vi "MultiAxisControl.vi"() -> ()   [LabVIEW 2020]
uses:
  <vilib>/Utility/config.llb/Read Key (I32).vi
  <vilib>/Utility/config.llb/Read Key (String).vi
  Recipe.vi
  <vilib>/Utility/config.llb/Write Key (I32).vi
  <vilib>/Utility/config.llb/Write Key (String).vi
  ConnectionData.vi
  ConnectionData_Write.vi
  <vilib>/Utility/config.llb/NI_LVConfig.lvlib
  SMCD14_lib.lvlib
panel:
  in  "StopAppBtn":bool caption="Close"
  in  "Recipe":bool
  in  "Chart":bool
  in  "DisconnectBtn":bool
  in  "ConnectBtn":bool
  out "AxesCount":i32=6
  out "AxisControlSubPanelsArray":refnum<vi>[](array[refnum])
  in  "error in (no error)":errorcluster
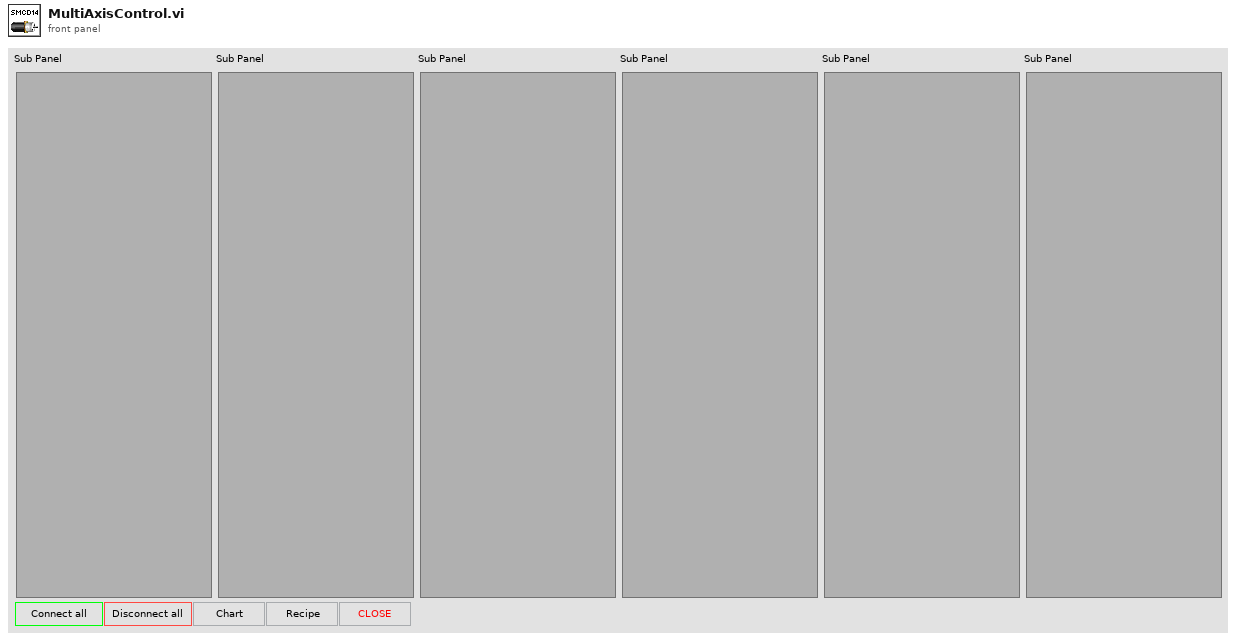
[diagram p1: front panel]
types:
  T1 = enum32{"Invalid", "Standard", "Closed", "Hidden", "Minimized", "Maximized"}
  T2 = typedef "NI_LVConfig.lvlib/Config Data RefNum.ctl" = refnum<k1>
  T3 = typedef "LVRectTypeDef.ctl" = cluster{"Left":i16, "Top":i16, "Right":i16, "Bottom":i16}
  T4 = enum32{"Bad", "Idle", "Run top level", "Running"}
  T5 = typedef "SMCD14_lib.lvlib/ConnectionData_typedef.ctl" = cluster{"DeviceIDCtrl":u16, "ProtocolCtrl":enum16{"Modbus RTU", "Modbus TCP", ""}, "COMportCtrl":refnum<visa-resource-name>, "IPCtrl":string, "serial master instance":refnum<class "Modbus Master.lvclass">, "ConnectionStatusIndicator":bool}
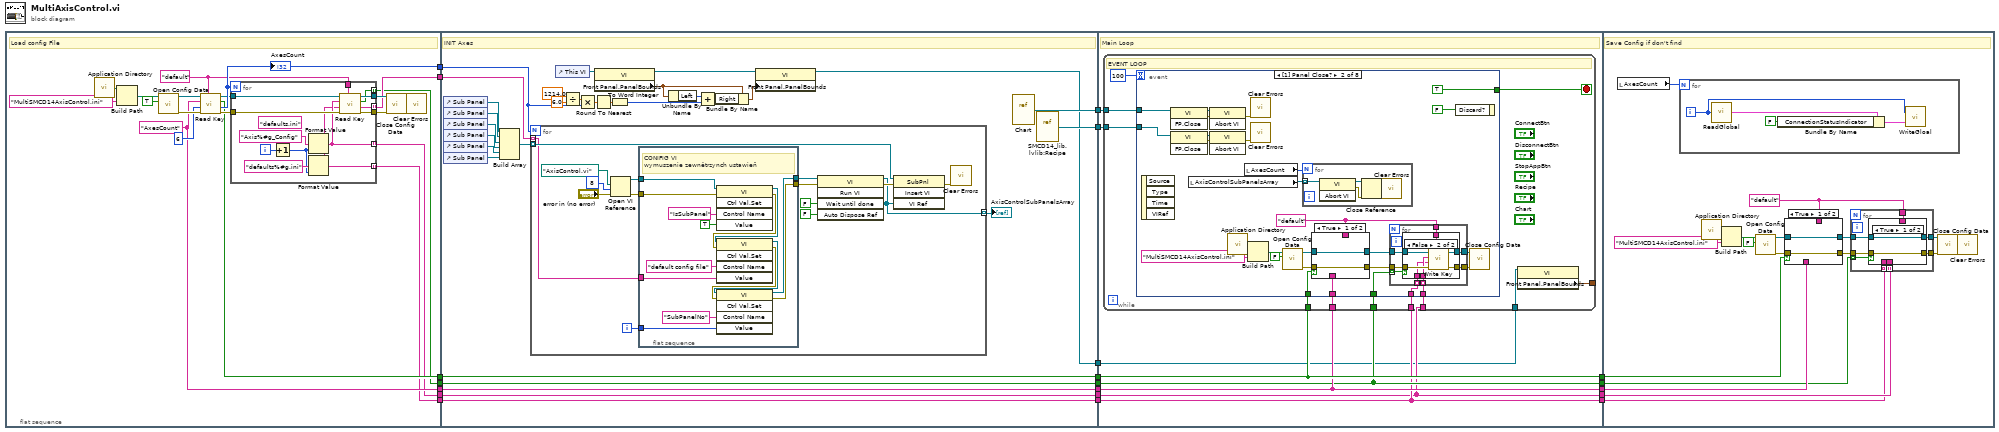
[diagram p0: block diagram]
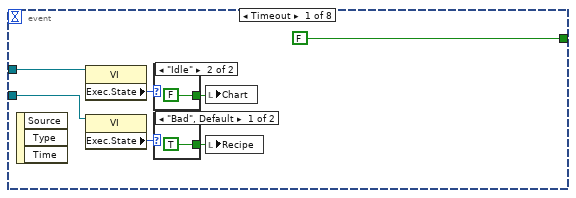
[diagram p2: hidden frame]
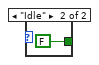
[diagram p3: hidden frame]
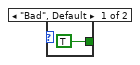
[diagram p4: hidden frame]
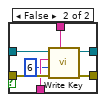
[diagram p6: hidden frame]
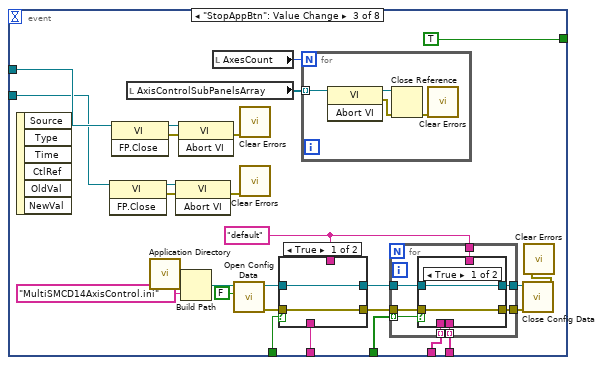
[diagram p7: hidden frame]
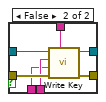
[diagram p8: hidden frame]
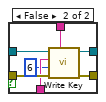
[diagram p9: hidden frame]
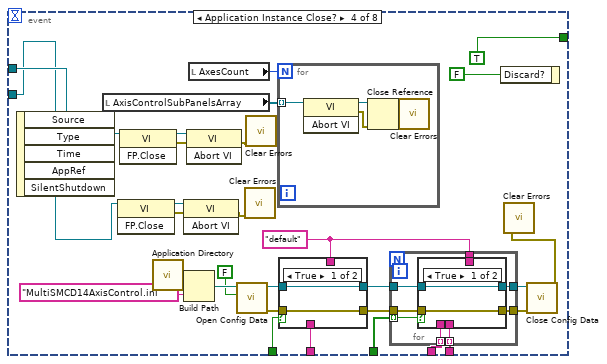
[diagram p10: hidden frame]
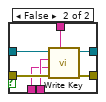
[diagram p11: hidden frame]
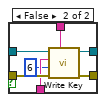
[diagram p12: hidden frame]
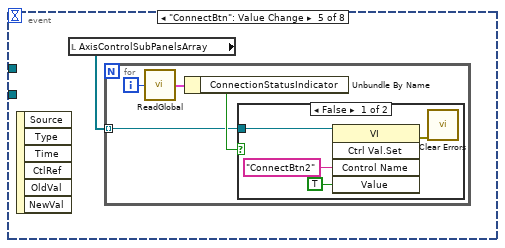
[diagram p13: hidden frame]
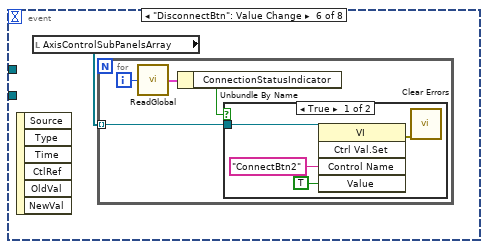
[diagram p15: hidden frame]
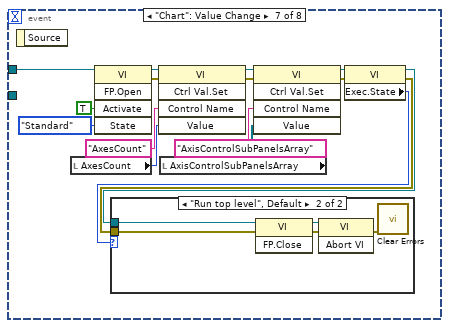
[diagram p17: hidden frame]
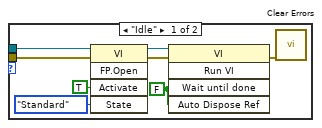
[diagram p18: hidden frame]
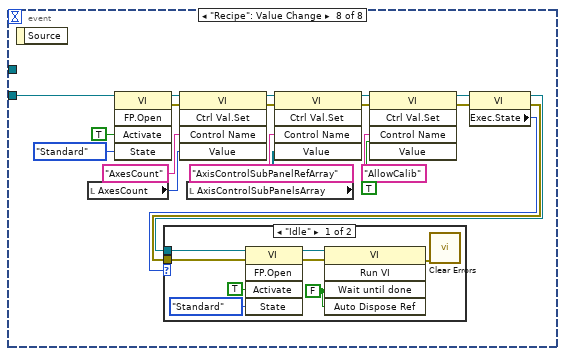
[diagram p19: hidden frame]
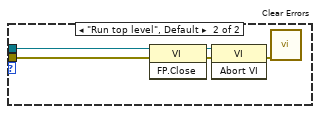
[diagram p20: hidden frame]
diagram:
  n1 = flat-sequence {
    tunnel: [w33] -> w20
    tunnel: [w27] -> w19
    tunnel: [w26] -> w18
    tunnel: [w25] -> w17
    tunnel: [w24] -> w12
    tunnel: [w23] -> w11
    tunnel: [w22] -> w10
    tunnel: w20 -> [w68]
    tunnel: w19 -> [w80]
    tunnel: w18 -> [w79]
    tunnel: w17 -> [w78]
    tunnel: [w79] -> w16
    tunnel: [w78] -> w15
    tunnel: w12 -> [w77]
    tunnel: w11 -> [w76]
    tunnel: w10 -> [w75]
    tunnel: [w77] -> w9
    tunnel: [w76] -> w8
    tunnel: [w75] -> w7
    tunnel: [w74] -> w3
    tunnel: [w73] -> w2
    tunnel: [w54] -> w1
    tunnel: w16 -> [w119]
    tunnel: w15 -> [w117]
    tunnel: [w119] -> w14
    tunnel: [w117] -> w13
    tunnel: w9 -> [w118]
    tunnel: w8 -> [w115]
    tunnel: w7 -> [w116]
    tunnel: [w118] -> w6
    tunnel: [w115] -> w5
    tunnel: [w116] -> w4
    tunnel: w3 -> [w114]
    tunnel: w2 -> [w113]
    tunnel: w1 -> [w112]
    tunnel: w14 -> [w407]
    tunnel: w13 -> [w404]
    tunnel: w6 -> [w408]
    tunnel: w5 -> [w406]
    tunnel: w4 -> [w405]
    frame #0 {
      w24 = "AxesCount" ("key")
      w30 = "default" ("section")
      # "Load config File"
      n2 = call <vilib>:"Application Directory.vi"() -> ("Application Directory"=w39:path)
      n3 = Build Path(base path=w39, name or relative path="MultiSMCD14AxisControl.ini") -> (appended path=w35:path)
      n4 = call <vilib>:"Open Config Data.vi"("create file if necessary (T)"=TRUE, "configuration file path"=w35) -> ("error out"=w36:errorcluster, "refnum"=w37:T2)  [unwired: 7 in, 1 out]
      n5 = call-poly <vilib>:"Read Key.vi"("section"=w30, "error in (no error)"=w36, "default value"=6, "key"=w24, "refnum"=w37) -> ("error out"=w31:errorcluster, "value"=w33:i32, "found?"=w26:bool, "refnum out"=w32:T2)  [unwired: 3 in]
      "AxesCount" <- w33
      n6 = for {
        N: w33 -> [_]
        tunnel: w32 -> [w51]
        tunnel: w31 -> [w50]
        tunnel: [w49] -> w29
        tunnel: [w48] -> w28
        tunnel: [w47] -> w27 mode=indexing
        tunnel: w30 -> [w46]
        tunnel: [w43] -> w25 mode=indexing
        tunnel: [w42] -> w23 mode=indexing
        tunnel: [w41] -> w22 mode=indexing
        i -> [w53]
        (unwired) "defaults.ini" ("default value")
        n7 = Increment(x=w53) -> (x+1=w44:i32)
        n8 = Format Value(format string="Axis%#g_Config" ("key"), value (0)=w44) -> (output string=w42:string)  [unwired: 1 in]
        n9 = Format Value(format string="defaults%#g.ini" ("default value"), value (0)=w44) -> (output string=w41:string)  [unwired: 1 in]
        n10 = call-poly <vilib>:"Read Key.vi"("section"=w46, "error in (no error)"=w50, "default value"=w41, "key"=w42, "refnum"=w51) -> ("error out"=w48:errorcluster, "value"=w47:string, "found?"=w43:bool, "refnum out"=w49:T2)  [unwired: 3 in]
      }
      n11 = call <vilib>:"Close Config Data.vi"("error in (no error)"=w28, "refnum"=w29) -> ("error out"=w21:errorcluster)  [unwired: 8 in, 1 out]
      n12 = call <vilib>:"Clear Errors.vi"("error in (no error)"=w21) -> ()  [unwired: 5 in, 2 out]
    }
    frame #1 {
      # "INIT Axes"
      n13 = control-ref of="Sub Panel"() -> (w60:refnum<vi>)
      n14 = control-ref of="Sub Panel"() -> (w59:refnum<vi>)
      n15 = control-ref of="Sub Panel"() -> (w58:refnum<vi>)
      n16 = control-ref of="Sub Panel"() -> (w57:refnum<vi>)
      n17 = control-ref of="Sub Panel"() -> (w56:refnum<vi>)
      n18 = control-ref of="Sub Panel"() -> (w55:refnum<vi>)
      n19 = Build Array(w60, w59, w58, w57, w56, w55) -> (w81:refnum<vi>[])
      n20 = for {
        N: w68 -> [_]
        tunnel: w81 -> [w94] mode=indexing
        tunnel: [w84] -> w82 mode=indexing
        tunnel: w80 -> [w86] mode=indexing
        i -> [w85]
        n21 = Open VI Reference(vi path=path "AxisControl.vi", options=8, error in (no error)="error in (no error)") -> (vi reference=w88:refnum<vi>, error out=w87:errorcluster)  [unwired: 3 in]
        n22 = flat-sequence {
          tunnel: w88 -> [w109]
          tunnel: [w100] -> w95
          tunnel: w87 -> [w108]
          tunnel: [w101] -> w93
          tunnel: w86 -> [w104]
          tunnel: w85 -> [w103]
          frame #0 {
            # "CONIFIG VI\nwymuszenie zewnêtrzynch ustawieñ"
            n23 = invoke class="VI" method="Ctrl Val.Set"(reference=w109, error in=w108, "Control Name"="IsSubPanel", "Value"=TRUE) -> (reference out=w106:refnum<vi>, error out=w105:errorcluster)  [unwired: 1 in, 3 out]
            n24 = invoke class="VI" method="Ctrl Val.Set"(reference=w106, error in=w105, "Control Name"="default config file", "Value"=w104) -> (reference out=w99:refnum<vi>, error out=w98:errorcluster)  [unwired: 1 in, 3 out]
            n25 = invoke class="VI" method="Ctrl Val.Set"(reference=w99, error in=w98, "Control Name"="SubPanelNo", "Value"=w103) -> (reference out=w101:refnum<vi>, error out=w100:errorcluster)  [unwired: 1 in, 3 out]
          }
        }
        n26 = invoke class="VI" method="Run VI"(reference=w93, error in=w95, "Wait until done"=FALSE ("Wait Until Done"), "Auto Dispose Ref"=FALSE ("Auto Dispose Reference")) -> (reference out=w84:refnum<vi>, error out=w92:errorcluster)  [unwired: 1 in, 3 out]
        n27 = invoke class="SubPnl" method="Insert VI"(reference=w94, error in=w92, "VI Ref"=w84) -> (error out=w83:errorcluster)  [unwired: 1 in, 3 out]
        n28 = call <vilib>:"Clear Errors.vi"("error in (no error)"=w83) -> ()  [unwired: 5 in, 2 out]
      }
      "AxisControlSubPanelsArray" <- w82
      n29 = control-ref of="This VI"() -> (w72:refnum<vi>)
      n30 = Divide(x=1214.0, y=6.0) -> (x/y=w69:dbl)
      n31 = Multiply(x=w69, y=w68) -> (x*y=w67:dbl)
      n32 = Round To Nearest(number=w67) -> (nearest integer value=w66:dbl)
      n33 = property class="VI"(reference=w72) -> ("Front Panel.PanelBounds"=w64:T3)  [unwired: 1 in, 2 out]
      n34 = To Word Integer(number=w66) -> (16bit integer=w62:i16)
      n35 = Unbundle By Name(w64) -> ("Left"=w61:i16)
      n36 = Add(x=w61, y=w62) -> (x+y=w63:i16)
      n37 = Bundle By Name(cluster=w64, "Right"=w63) -> (w65:T3)
      n38 = property class="VI"(reference=w72, "Front Panel.PanelBounds"=w65) -> (reference out=w54:refnum<vi>)  [unwired: 1 in, 1 out]
      n39 = vi-ref "Chart.vi"() -> (w74:refnum<vi>)
      n40 = vi-ref "SMCD14_lib.lvlib:Recipe.vi"() -> (w73:refnum<vi>)
    }
    frame #2 {
      # "Main Loop"
      n41 = while {
        tunnel: w119 -> [w128]
        tunnel: w118 -> [w127]
        tunnel: w117 -> [w126]
        tunnel: w116 -> [w125]
        tunnel: w115 -> [w124]
        tunnel: w114 -> [w123]
        tunnel: w113 -> [w122]
        tunnel: [w121] -> _
        tunnel: w112 -> [w120]
        stop <- w129 stop-if-true
        # "EVENT LOOP"
        n42 = event shown="[1] Panel Close?" {
          selector: _ -> [_ _ _ _ _ _ _ _]
          dyn-events: _ -> [_ _ _ _ _ _ _ _]
          timeout: 100 -> [_ _ _ _ _ _ _ _]
          tunnel: [FALSE ("Discard?") TRUE ("Discard?") TRUE ("Discard?") TRUE ("Discard?") _ _ _ _] -> w129
          tunnel: w128 -> [_ w154 w213 w275 _ _ _ _]
          tunnel: w127 -> [_ w153 w212 w274 _ _ _ _]
          tunnel: w126 -> [_ w152 w211 w273 _ _ _ _]
          tunnel: w125 -> [_ w151 w210 w272 _ _ _ _]
          tunnel: w124 -> [_ w150 w209 w271 _ _ _ _]
          tunnel: w123 -> [w136 w149 w208 w262 _ _ w344 _]
          tunnel: w122 -> [w132 w146 w205 w261 _ _ _ w371]
          event Timeout {
            n43 = event-data() -> ()  [unwired: 1 in, 3 out]
            n44 = property class="VI"(reference=w136) -> ("Exec.State"=w135:T4)  [unwired: 1 in, 2 out]
            n45 = property class="VI"(reference=w132) -> ("Exec.State"=w133:T4)  [unwired: 1 in, 2 out]
            n46 = case shown="\"Idle\"" w135 {
              tunnel: [TRUE ("Chart") FALSE ("Chart")] -> w134
              frame "Bad", Default {
              }
              frame "Idle" {
              }
            }
            n47 = case shown="\"Bad\", Default" w133 {
              tunnel: [TRUE ("Chart") FALSE ("Chart")] -> w131
              frame "Bad", Default {
              }
              frame "Idle" {
              }
            }
            n48 = local write "Chart"(w134) -> ()
            n49 = local write "Recipe"(w131) -> ()
          }
          event Panel Close? {
            w159 = "default" ("section")
            n50 = event-data() -> ()  [unwired: 1 in, 4 out]
            n51 = invoke class="VI" method="FP.Close"(reference=w149) -> (reference out=w148:refnum<vi>, error out=w145:errorcluster)  [unwired: 2 in, 1 out]
            n52 = invoke class="VI" method="FP.Close"(reference=w146) -> (reference out=w147:refnum<vi>, error out=w144:errorcluster)  [unwired: 2 in, 1 out]
            n53 = local read "AxisControlSubPanelsArray"() -> (w169:refnum<vi>[])
            n54 = invoke class="VI" method="Abort VI"(reference=w148, error in=w145) -> (error out=w143:errorcluster)  [unwired: 1 in, 2 out]
            n55 = invoke class="VI" method="Abort VI"(reference=w147, error in=w144) -> (error out=w142:errorcluster)  [unwired: 1 in, 2 out]
            n56 = call <vilib>:"Application Directory.vi"() -> ("Application Directory"=w162:path)
            n57 = local read "AxesCount"() -> (w167:i32)
            n58 = Build Path(base path=w162, name or relative path="MultiSMCD14AxisControl.ini") -> (appended path=w163:path)
            n59 = call <vilib>:"Clear Errors.vi"("error in (no error)"=w143) -> ()  [unwired: 5 in, 2 out]
            n60 = call <vilib>:"Clear Errors.vi"("error in (no error)"=w142) -> ()  [unwired: 5 in, 2 out]
            n61 = call <vilib>:"Open Config Data.vi"("create file if necessary (T)"=FALSE, "configuration file path"=w163) -> ("error out"=w165:errorcluster, "refnum"=w164:T2)  [unwired: 7 in, 1 out]
            n62 = for {
              N: w167 -> [_]
              tunnel: w169 -> [w199] mode=indexing
              n63 = invoke class="VI" method="Abort VI"(reference=w199) -> (reference out=w198:refnum<vi>, error out=w197:errorcluster)  [unwired: 2 in, 1 out]
              n64 = Close Reference(reference=w198, error in (no error)=w197) -> (error out=w196:errorcluster)
              n65 = call <vilib>:"Clear Errors.vi"("error in (no error)"=w196) -> ()  [unwired: 5 in, 2 out]
            }
            n66 = case shown="True" w154 {
              tunnel: [w187 w195] -> w157
              tunnel: [w188 w194] -> w158
              tunnel: w165 -> [w187 w193]
              tunnel: w164 -> [w188 w192]
              tunnel: w153 -> [_ w191]
              tunnel: w159 -> [_ w189]
              frame True {
              }
              frame False {
                n67 = call-poly <vilib>:"Write Key.vi"("section"=w189, "error in (no error)"=w193, "value"=6, "key"=w191, "refnum"=w192) -> ("error out"=w195:errorcluster, "refnum out"=w194:T2)  [unwired: 4 in, 1 out]
              }
            }
            n68 = for {
              tunnel: w150 -> [w177] mode=indexing
              tunnel: w151 -> [w176] mode=indexing
              tunnel: w152 -> [w170] mode=indexing
              tunnel: w159 -> [w175]
              tunnel: w158 -> [w174]
              tunnel: w157 -> [w173]
              tunnel: [w172] -> w156
              tunnel: [w171] -> w155
              n69 = case shown="False" w170 {
                tunnel: [w178 w186] -> w171
                tunnel: [w179 w185] -> w172
                tunnel: w173 -> [w178 w184]
                tunnel: w174 -> [w179 w183]
                tunnel: w177 -> [_ w182]
                tunnel: w175 -> [_ w181]
                tunnel: w176 -> [_ w180]
                frame True {
                }
                frame False {
                  n70 = call-poly <vilib>:"Write Key.vi"("section"=w181, "error in (no error)"=w184, "value"=w180, "key"=w182, "refnum"=w183) -> ("error out"=w186:errorcluster, "refnum out"=w185:T2)  [unwired: 4 in, 1 out]
                }
              }
            }
            n71 = event-data("Discard?"=FALSE) -> ()  [unwired: 1 in, 1 out]
            n72 = call <vilib>:"Close Config Data.vi"("error in (no error)"=w155, "refnum"=w156) -> ()  [unwired: 8 in, 2 out]
          }
          event "StopAppBtn": Value Change {
            w218 = "default" ("section")
            n73 = event-data() -> ()  [unwired: 1 in, 6 out]
            n74 = invoke class="VI" method="FP.Close"(reference=w205) -> (reference out=w206:refnum<vi>, error out=w203:errorcluster)  [unwired: 2 in, 1 out]
            n75 = invoke class="VI" method="FP.Close"(reference=w208) -> (reference out=w207:refnum<vi>, error out=w204:errorcluster)  [unwired: 2 in, 1 out]
            n76 = local read "AxisControlSubPanelsArray"() -> (w227:refnum<vi>[])
            n77 = call <vilib>:"Application Directory.vi"() -> ("Application Directory"=w221:path)
            n78 = invoke class="VI" method="Abort VI"(reference=w206, error in=w203) -> (error out=w202:errorcluster)  [unwired: 1 in, 2 out]
            n79 = invoke class="VI" method="Abort VI"(reference=w207, error in=w204) -> (error out=w201:errorcluster)  [unwired: 1 in, 2 out]
            n80 = Build Path(base path=w221, name or relative path="MultiSMCD14AxisControl.ini") -> (appended path=w222:path)
            n81 = local read "AxesCount"() -> (w226:i32)
            n82 = call <vilib>:"Open Config Data.vi"("create file if necessary (T)"=FALSE, "configuration file path"=w222) -> ("error out"=w224:errorcluster, "refnum"=w223:T2)  [unwired: 7 in, 1 out]
            n83 = call <vilib>:"Clear Errors.vi"("error in (no error)"=w201) -> ()  [unwired: 5 in, 2 out]
            n84 = call <vilib>:"Clear Errors.vi"("error in (no error)"=w202) -> ()  [unwired: 5 in, 2 out]
            n85 = case shown="True" w213 {
              tunnel: [w245 w253] -> w216
              tunnel: [w246 w252] -> w217
              tunnel: w224 -> [w245 w251]
              tunnel: w223 -> [w246 w250]
              tunnel: w212 -> [_ w249]
              tunnel: w218 -> [_ w247]
              frame True {
              }
              frame False {
                n86 = call-poly <vilib>:"Write Key.vi"("section"=w247, "error in (no error)"=w251, "value"=6, "key"=w249, "refnum"=w250) -> ("error out"=w253:errorcluster, "refnum out"=w252:T2)  [unwired: 4 in, 1 out]
              }
            }
            n87 = for {
              N: w226 -> [_]
              tunnel: w227 -> [w257] mode=indexing
              n88 = invoke class="VI" method="Abort VI"(reference=w257) -> (reference out=w256:refnum<vi>, error out=w255:errorcluster)  [unwired: 2 in, 1 out]
              n89 = Close Reference(reference=w256, error in (no error)=w255) -> (error out=w254:errorcluster)
              n90 = call <vilib>:"Clear Errors.vi"("error in (no error)"=w254) -> ()  [unwired: 5 in, 2 out]
            }
            n91 = for {
              tunnel: w209 -> [w235] mode=indexing
              tunnel: w210 -> [w234] mode=indexing
              tunnel: w211 -> [w228] mode=indexing
              tunnel: w218 -> [w233]
              tunnel: w217 -> [w232]
              tunnel: w216 -> [w231]
              tunnel: [w230] -> w215
              tunnel: [w229] -> w214
              n92 = case shown="True" w228 {
                tunnel: [w236 w244] -> w229
                tunnel: [w237 w243] -> w230
                tunnel: w231 -> [w236 w242]
                tunnel: w232 -> [w237 w241]
                tunnel: w235 -> [_ w240]
                tunnel: w233 -> [_ w239]
                tunnel: w234 -> [_ w238]
                frame True {
                }
                frame False {
                  n93 = call-poly <vilib>:"Write Key.vi"("section"=w239, "error in (no error)"=w242, "value"=w238, "key"=w240, "refnum"=w241) -> ("error out"=w244:errorcluster, "refnum out"=w243:T2)  [unwired: 4 in, 1 out]
                }
              }
            }
            n94 = call <vilib>:"Close Config Data.vi"("error in (no error)"=w214, "refnum"=w215) -> ("error out"=w200:errorcluster)  [unwired: 8 in, 1 out]
            n95 = call <vilib>:"Clear Errors.vi"("error in (no error)"=w200) -> ()  [unwired: 5 in, 2 out]
          }
          event Application Instance Close? {
            w280 = "default" ("section")
            n96 = event-data() -> ()  [unwired: 1 in, 5 out]
            n97 = local read "AxisControlSubPanelsArray"() -> (w264:refnum<vi>[])
            n98 = invoke class="VI" method="FP.Close"(reference=w261) -> (reference out=w267:refnum<vi>, error out=w269:errorcluster)  [unwired: 2 in, 1 out]
            n99 = invoke class="VI" method="FP.Close"(reference=w262) -> (reference out=w266:refnum<vi>, error out=w268:errorcluster)  [unwired: 2 in, 1 out]
            n100 = call <vilib>:"Application Directory.vi"() -> ("Application Directory"=w283:path)
            n101 = invoke class="VI" method="Abort VI"(reference=w267, error in=w269) -> (error out=w259:errorcluster)  [unwired: 1 in, 2 out]
            n102 = Build Path(base path=w283, name or relative path="MultiSMCD14AxisControl.ini") -> (appended path=w284:path)
            n103 = invoke class="VI" method="Abort VI"(reference=w266, error in=w268) -> (error out=w260:errorcluster)  [unwired: 1 in, 2 out]
            n104 = local read "AxesCount"() -> (w265:i32)
            n105 = call <vilib>:"Open Config Data.vi"("create file if necessary (T)"=FALSE, "configuration file path"=w284) -> ("error out"=w286:errorcluster, "refnum"=w285:T2)  [unwired: 7 in, 1 out]
            n106 = call <vilib>:"Clear Errors.vi"("error in (no error)"=w259) -> ()  [unwired: 5 in, 2 out]
            n107 = call <vilib>:"Clear Errors.vi"("error in (no error)"=w260) -> ()  [unwired: 5 in, 2 out]
            n108 = for {
              N: w265 -> [_]
              tunnel: w264 -> [w290] mode=indexing
              n109 = invoke class="VI" method="Abort VI"(reference=w290) -> (reference out=w289:refnum<vi>, error out=w288:errorcluster)  [unwired: 2 in, 1 out]
              n110 = Close Reference(reference=w289, error in (no error)=w288) -> (error out=w287:errorcluster)
              n111 = call <vilib>:"Clear Errors.vi"("error in (no error)"=w287) -> ()  [unwired: 5 in, 2 out]
            }
            n112 = case shown="True" w275 {
              tunnel: [w308 w316] -> w278
              tunnel: [w309 w315] -> w279
              tunnel: w286 -> [w308 w314]
              tunnel: w285 -> [w309 w313]
              tunnel: w274 -> [_ w312]
              tunnel: w280 -> [_ w310]
              frame True {
              }
              frame False {
                n113 = call-poly <vilib>:"Write Key.vi"("section"=w310, "error in (no error)"=w314, "value"=6, "key"=w312, "refnum"=w313) -> ("error out"=w316:errorcluster, "refnum out"=w315:T2)  [unwired: 4 in, 1 out]
              }
            }
            n114 = for {
              tunnel: w271 -> [w298] mode=indexing
              tunnel: w272 -> [w297] mode=indexing
              tunnel: w273 -> [w291] mode=indexing
              tunnel: w280 -> [w296]
              tunnel: w279 -> [w295]
              tunnel: w278 -> [w294]
              tunnel: [w293] -> w277
              tunnel: [w292] -> w276
              n115 = case shown="True" w291 {
                tunnel: [w299 w307] -> w292
                tunnel: [w300 w306] -> w293
                tunnel: w294 -> [w299 w305]
                tunnel: w295 -> [w300 w304]
                tunnel: w298 -> [_ w303]
                tunnel: w296 -> [_ w302]
                tunnel: w297 -> [_ w301]
                frame True {
                }
                frame False {
                  n116 = call-poly <vilib>:"Write Key.vi"("section"=w302, "error in (no error)"=w305, "value"=w301, "key"=w303, "refnum"=w304) -> ("error out"=w307:errorcluster, "refnum out"=w306:T2)  [unwired: 4 in, 1 out]
                }
              }
            }
            n117 = event-data("Discard?"=FALSE) -> ()  [unwired: 1 in, 1 out]
            n118 = call <vilib>:"Close Config Data.vi"("error in (no error)"=w276, "refnum"=w277) -> ("error out"=w258:errorcluster)  [unwired: 8 in, 1 out]
            n119 = call <vilib>:"Clear Errors.vi"("error in (no error)"=w258) -> ()  [unwired: 5 in, 2 out]
          }
          event "ConnectBtn": Value Change {
            n120 = event-data() -> ()  [unwired: 1 in, 6 out]
            n121 = local read "AxisControlSubPanelsArray"() -> (w317:refnum<vi>[])
            n122 = for {
              tunnel: w317 -> [w318] mode=indexing
              i -> [w320]
              n123 = call-poly "ReadGlobal.vi"("AxisNo"=w320) -> ("ConnectionDataOUT"=w321:T5)
              n124 = Unbundle By Name(w321) -> ("ConnectionStatusIndicator"=w319:bool)
              n125 = case shown="False" w319 {
                tunnel: w318 -> [w323 _]
                frame False {
                  n126 = invoke class="VI" method="Ctrl Val.Set"(reference=w323, "Control Name"="ConnectBtn2", "Value"=TRUE) -> (error out=w322:errorcluster)  [unwired: 2 in, 4 out]
                  n127 = call <vilib>:"Clear Errors.vi"("error in (no error)"=w322) -> ()  [unwired: 5 in, 2 out]
                }
                frame True {
                }
              }
            }
          }
          event "DisconnectBtn": Value Change {
            n128 = event-data() -> ()  [unwired: 1 in, 6 out]
            n129 = local read "AxisControlSubPanelsArray"() -> (w326:refnum<vi>[])
            n130 = for {
              tunnel: w326 -> [w327] mode=indexing
              i -> [w329]
              n131 = call-poly "ReadGlobal.vi"("AxisNo"=w329) -> ("ConnectionDataOUT"=w330:T5)
              n132 = Unbundle By Name(w330) -> ("ConnectionStatusIndicator"=w328:bool)
              n133 = case shown="True" w328 {
                tunnel: w327 -> [w332 _]
                frame True {
                  n134 = invoke class="VI" method="Ctrl Val.Set"(reference=w332, "Control Name"="ConnectBtn2", "Value"=TRUE) -> (error out=w331:errorcluster)  [unwired: 2 in, 4 out]
                  n135 = call <vilib>:"Clear Errors.vi"("error in (no error)"=w331) -> ()  [unwired: 5 in, 2 out]
                }
                frame False {
                }
              }
            }
          }
          event "Chart": Value Change {
            n136 = event-data() -> ()  [unwired: 1 in, 1 out]
            n137 = local read "AxesCount"() -> (w349:i32)
            n138 = invoke class="VI" method="FP.Open"(reference=w344, "Activate"=TRUE ("Activate?"), "State"=T1."Standard") -> (reference out=w348:refnum<vi>, error out=w347:errorcluster)  [unwired: 2 in, 3 out]
            n139 = invoke class="VI" method="Ctrl Val.Set"(reference=w348, error in=w347, "Control Name"="AxesCount", "Value"=w349) -> (reference out=w339:refnum<vi>, error out=w338:errorcluster)  [unwired: 1 in, 3 out]
            n140 = local read "AxisControlSubPanelsArray"() -> (w340:refnum<vi>[])
            n141 = invoke class="VI" method="Ctrl Val.Set"(reference=w339, error in=w338, "Control Name"="AxisControlSubPanelsArray", "Value"=w340) -> (reference out=w337:refnum<vi>, error out=w336:errorcluster)  [unwired: 1 in, 3 out]
            n142 = property class="VI"(reference=w337, error in=w336) -> (reference out=w343:refnum<vi>, error out=w342:errorcluster, "Exec.State"=w335:T4)
            n143 = case shown="\"Run top level\", Default" w335 {
              tunnel: w343 -> [w352 w363]
              tunnel: w342 -> [w351 w362]
              frame "Idle" {
                w358 = FALSE ("Activate?")
                n144 = invoke class="VI" method="FP.Open"(reference=w352, error in=w351, "Activate"=TRUE ("Activate?"), "State"=T1."Standard") -> (reference out=w356:refnum<vi>, error out=w357:errorcluster)  [unwired: 1 in, 3 out]
                n145 = invoke class="VI" method="Run VI"(reference=w356, error in=w357, "Wait until done"=w358, "Auto Dispose Ref"=w358) -> (error out=w353:errorcluster)  [unwired: 1 in, 4 out]
                n146 = call <vilib>:"Clear Errors.vi"("error in (no error)"=w353) -> ()  [unwired: 5 in, 2 out]
              }
              frame "Run top level", Default {
                n147 = invoke class="VI" method="FP.Close"(reference=w363, error in=w362) -> (reference out=w361:refnum<vi>, error out=w360:errorcluster)  [unwired: 1 in, 1 out]
                n148 = invoke class="VI" method="Abort VI"(reference=w361, error in=w360) -> (error out=w359:errorcluster)  [unwired: 1 in, 2 out]
                n149 = call <vilib>:"Clear Errors.vi"("error in (no error)"=w359) -> ()  [unwired: 5 in, 2 out]
              }
            }
          }
          event "Recipe": Value Change {
            n150 = event-data() -> ()  [unwired: 1 in, 1 out]
            n151 = local read "AxesCount"() -> (w383:i32)
            n152 = invoke class="VI" method="FP.Open"(reference=w371, "Activate"=TRUE ("Activate?"), "State"=T1."Standard") -> (reference out=w382:refnum<vi>, error out=w381:errorcluster)  [unwired: 2 in, 3 out]
            n153 = invoke class="VI" method="Ctrl Val.Set"(reference=w382, error in=w381, "Control Name"="AxesCount", "Value"=w383) -> (reference out=w373:refnum<vi>, error out=w372:errorcluster)  [unwired: 1 in, 3 out]
            n154 = local read "AxisControlSubPanelsArray"() -> (w374:refnum<vi>[])
            n155 = invoke class="VI" method="Ctrl Val.Set"(reference=w373, error in=w372, "Control Name"="AxisControlSubPanelRefArray", "Value"=w374) -> (reference out=w369:refnum<vi>, error out=w368:errorcluster)  [unwired: 1 in, 3 out]
            n156 = invoke class="VI" method="Ctrl Val.Set"(reference=w369, error in=w368, "Control Name"="AllowCalib", "Value"=TRUE) -> (reference out=w367:refnum<vi>, error out=w366:errorcluster)  [unwired: 1 in, 3 out]
            n157 = property class="VI"(reference=w367, error in=w366) -> (reference out=w378:refnum<vi>, error out=w376:errorcluster, "Exec.State"=w377:T4)
            n158 = case shown="\"Idle\"" w377 {
              tunnel: w378 -> [w386 w396]
              tunnel: w376 -> [w385 w395]
              frame "Idle" {
                w391 = FALSE ("Activate?")
                n159 = invoke class="VI" method="FP.Open"(reference=w386, error in=w385, "Activate"=TRUE ("Activate?"), "State"=T1."Standard") -> (reference out=w389:refnum<vi>, error out=w390:errorcluster)  [unwired: 1 in, 3 out]
                n160 = invoke class="VI" method="Run VI"(reference=w389, error in=w390, "Wait until done"=w391, "Auto Dispose Ref"=w391) -> (error out=w384:errorcluster)  [unwired: 1 in, 4 out]
                n161 = call <vilib>:"Clear Errors.vi"("error in (no error)"=w384) -> ()  [unwired: 5 in, 2 out]
              }
              frame "Run top level", Default {
                n162 = invoke class="VI" method="FP.Close"(reference=w396, error in=w395) -> (reference out=w394:refnum<vi>, error out=w393:errorcluster)  [unwired: 1 in, 1 out]
                n163 = invoke class="VI" method="Abort VI"(reference=w394, error in=w393) -> (error out=w392:errorcluster)  [unwired: 1 in, 2 out]
                n164 = call <vilib>:"Clear Errors.vi"("error in (no error)"=w392) -> ()  [unwired: 5 in, 2 out]
              }
            }
          }
        }
        n165 = property class="VI"(reference=w120) -> ("Front Panel.PanelBounds"=w121:T3)  [unwired: 1 in, 2 out]
      }
    }
    frame #3 {
      w403 = "default" ("section")
      # "Save Config if don't find"
      n166 = local read "AxesCount"() -> (w398:i32)
      n167 = for {
        N: w398 -> [_]
        i -> [w415]
        n168 = call-poly "ReadGlobal.vi"("AxisNo"=w415) -> ("ConnectionDataOUT"=w418:T5)
        n169 = Bundle By Name(cluster=w418, "ConnectionStatusIndicator"=FALSE) -> (w417:T5)
        n170 = call-poly "WriteGloal.vi"("ConnectionDataIN"=w417, "AxisNo"=w415) -> ()  [unwired: 1 in]
      }
      n171 = call <vilib>:"Application Directory.vi"() -> ("Application Directory"=w411:path)
      n172 = Build Path(base path=w411, name or relative path="MultiSMCD14AxisControl.ini") -> (appended path=w412:path)
      n173 = call <vilib>:"Open Config Data.vi"("create file if necessary (T)"=FALSE, "configuration file path"=w412) -> ("error out"=w414:errorcluster, "refnum"=w413:T2)  [unwired: 7 in, 1 out]
      n174 = case shown="True" w407 {
        tunnel: [w436 w444] -> w401
        tunnel: [w437 w443] -> w402
        tunnel: w414 -> [w436 w442]
        tunnel: w413 -> [w437 w441]
        tunnel: w408 -> [_ w440]
        tunnel: w403 -> [_ w438]
        frame True {
        }
        frame False {
          n175 = call-poly <vilib>:"Write Key.vi"("section"=w438, "error in (no error)"=w442, "value"=6, "key"=w440, "refnum"=w441) -> ("error out"=w444:errorcluster, "refnum out"=w443:T2)  [unwired: 4 in, 1 out]
        }
      }
      n176 = for {
        tunnel: w406 -> [w426] mode=indexing
        tunnel: w405 -> [w425] mode=indexing
        tunnel: w404 -> [w419] mode=indexing
        tunnel: w403 -> [w424]
        tunnel: w402 -> [w423]
        tunnel: w401 -> [w422]
        tunnel: [w421] -> w400
        tunnel: [w420] -> w399
        n177 = case shown="True" w419 {
          tunnel: [w427 w435] -> w420
          tunnel: [w428 w434] -> w421
          tunnel: w422 -> [w427 w433]
          tunnel: w423 -> [w428 w432]
          tunnel: w426 -> [_ w431]
          tunnel: w424 -> [_ w430]
          tunnel: w425 -> [_ w429]
          frame True {
          }
          frame False {
            n178 = call-poly <vilib>:"Write Key.vi"("section"=w430, "error in (no error)"=w433, "value"=w429, "key"=w431, "refnum"=w432) -> ("error out"=w435:errorcluster, "refnum out"=w434:T2)  [unwired: 4 in, 1 out]
          }
        }
      }
      n179 = call <vilib>:"Close Config Data.vi"("error in (no error)"=w399, "refnum"=w400) -> ("error out"=w397:errorcluster)  [unwired: 8 in, 1 out]
      n180 = call <vilib>:"Clear Errors.vi"("error in (no error)"=w397) -> ()  [unwired: 5 in, 2 out]
    }
  }
